vi "MAIN_CALLED_leerQR.vi"(8 "Error In":errorcluster, 11 "VISA resource name out":refnum<visa-resource-name>) -> (0 "Error Out":errorcluster)   [LabVIEW 2019]
uses:
  LVPROJ_CONFIG_ESTACION/Type_defs/Coordenadas_estacion.ctl
  LVPROJ_CREAR BANDEJAS/Type_defs/Data_Bandeja.ctl
  TYPE'S DEF/INPUT LECTURA_QR.ctl
  TYPE'S DEF/OUTPUTS_lecturaQR.ctl
  TYPE'S DEF/State_QR.ctl
  LVPROJ_MOVIMIENTO_CABEZAL/LABVIEW_MOVIMIENTO/MOVIMIENTO CABEZAL/Typedefs/Comandos.ctl
  LVPROJ_MOVIMIENTO_CABEZAL/LABVIEW_MOVIMIENTO/MOVIMIENTO CABEZAL/Typedefs/Estados_arduino.ctl
  <vilib>/Utility/error.llb/Error Cluster From Error Code.vi
  <vilib>/ErrorRing/Error Ring.xnode
  SHARED VI'S/SHARED VI'S.lvlib
panel:
  out "celda de comienzo leída":string
  out "datos leídos estacion":string
  out "trama datos enviada":string
  out "código leído?":bool
  out "read buffer 2":string
  out "caracter leido":string
  out "read buffer 3":string
  in  "Tab Control":T1(tab)
  in  "ENVIAR PARAMETROS DE LECTURA":bool
  in  "EXIT":bool
  in  "COMENZAR LECTURA":bool
  in  "LECTURA QR INPUT":T2={"COORD X"=0, "COORD  Y"=0, "NºASICS"=1, "SELECCIÓN DE BANDEJA"=enum."BANDEJA ENTRADA", "CONTEO QR"=0}
  out "INDICADORES DE TEST":T3
  out "EStado fsm":T4
  out "Configuracion Estación":T5={"Coordenadas_estacion"={"Coord.Bandeja entrada"={"Coord. X0 entrada"=0, "Coord. Y0 entrada "=0, "Altura Z entrada"=0}, "Coord.Bandeja OK"={"Coord. X0 OK"=0, "Coord. Y0 OK"=0, "Altura Z OK"=0}, "Coord.Bandeja entrada FAIL"={"Coord. X0 FAIL"=0, "Coord. Y0 FAIL"=0, "Altura Z FAIL"=0}, "Coord. Socket"={"Coord. X socket"=0, "Coord. Y socket"=0, "Altura Z socket"=0}}, "Nombre Bandeja"="", "Datos bandeja"={"Nº de columnas "=0, "Nº de filas "=0, "largo"=0, "ancho"=0, "nombre"="nombre", "Paso X (en mm)"=0.0, "Paso Y (en mm)"=0.0, "DISTANCIA SUELO A CHIP  "=0.0, "Nº de celdas totales"=0, "Distancia chips bandejas contiguas"=0.0}}
  out "FINAL QR?":bool
  out "QR pendientes":u32
  # "CELDA DE COMIENZO"
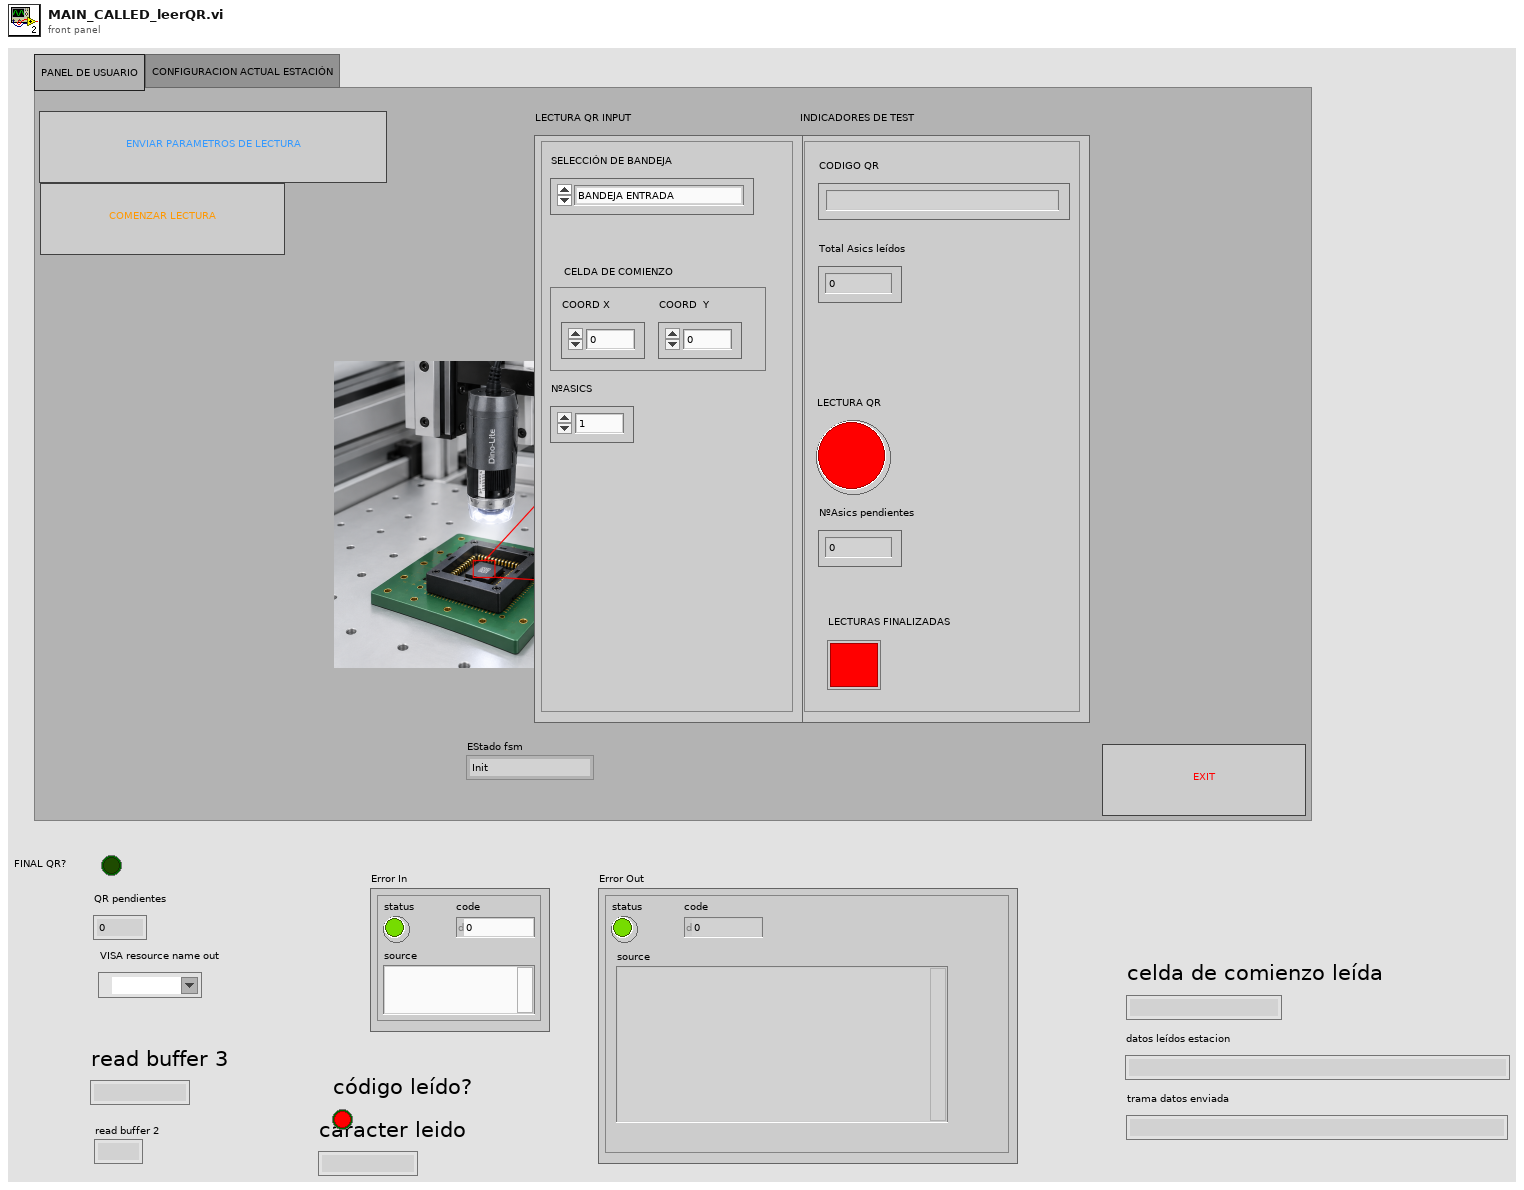
[diagram p1: front panel]
types:
  T1 = enum32{"PANEL DE USUARIO", "CONFIGURACION ACTUAL ESTACIÓN"}
  T2 = typedef "INPUT LECTURA_QR.ctl" = cluster{"COORD X":u16, "COORD  Y":u16, "NºASICS":u32, "SELECCIÓN DE BANDEJA":enum16{"BANDEJA ENTRADA", "BANDEJA OK", "BANDEJA NOK"}, "CONTEO QR":u32}
  T3 = typedef "OUTPUTS_lecturaQR.ctl" = cluster{"CODIGO QR":string, "LECTURA QR":bool, "LECTURAS FINALIZADAS":bool, "Total Asics leídos":u32, "NºAsics pendientes":u32}
  T4 = typedef "State_QR.ctl" = enum16{"Init", "Wait for Event", "Init refs", "Init com", "Config estacion", "Home", "Ping_Arduino", "Coge Asic", "Enviar_config_test", "Dejar Asic", "Leer QR", "Actualizar valores", "Enviar OK Arduino", "Final de lecturas?", "Terminar", "Exit", "Error?"}
  T5 = typedef "Configuracion_estación.ctl" = cluster{"Coordenadas_estacion":T6, "Nombre Bandeja":string, "Datos bandeja":T7}
  T6 = typedef "Coordenadas_estacion.ctl" = cluster{"Coord.Bandeja entrada":cluster{"Coord. X0 entrada":u32, "Coord. Y0 entrada ":u32, "Altura Z entrada":u32}, "Coord.Bandeja OK":cluster{"Coord. X0 OK":u32, "Coord. Y0 OK":u32, "Altura Z OK":u32}, "Coord.Bandeja entrada FAIL":cluster{"Coord. X0 FAIL":u32, "Coord. Y0 FAIL":u32, "Altura Z FAIL":u32}, "Coord. Socket":cluster{"Coord. X socket":u32, "Coord. Y socket":u32, "Altura Z socket":u32}}
  T7 = typedef "Data_Bandeja.ctl" = cluster{"Nº de columnas ":u32, "Nº de filas ":u32, "largo":u32, "ancho":u32, "nombre":string, "Paso X (en mm)":dbl, "Paso Y (en mm)":dbl, "DISTANCIA SUELO A CHIP  ":dbl, "Nº de celdas totales":u16, "Distancia chips bandejas contiguas":dbl}
  T8 = typedef "Comandos.ctl" = enum16{"H", "FH", "FM", "FI", "FX", "FY", "FZ", "I", "OK"}
  T9 = typedef "Estados_arduino.ctl" = enum16{"2", "3", "4", "5", "6", "7", "9", "8"}
  T10 = enum16{"BANDEJA ENTRADA", "BANDEJA OK", "BANDEJA NOK"}
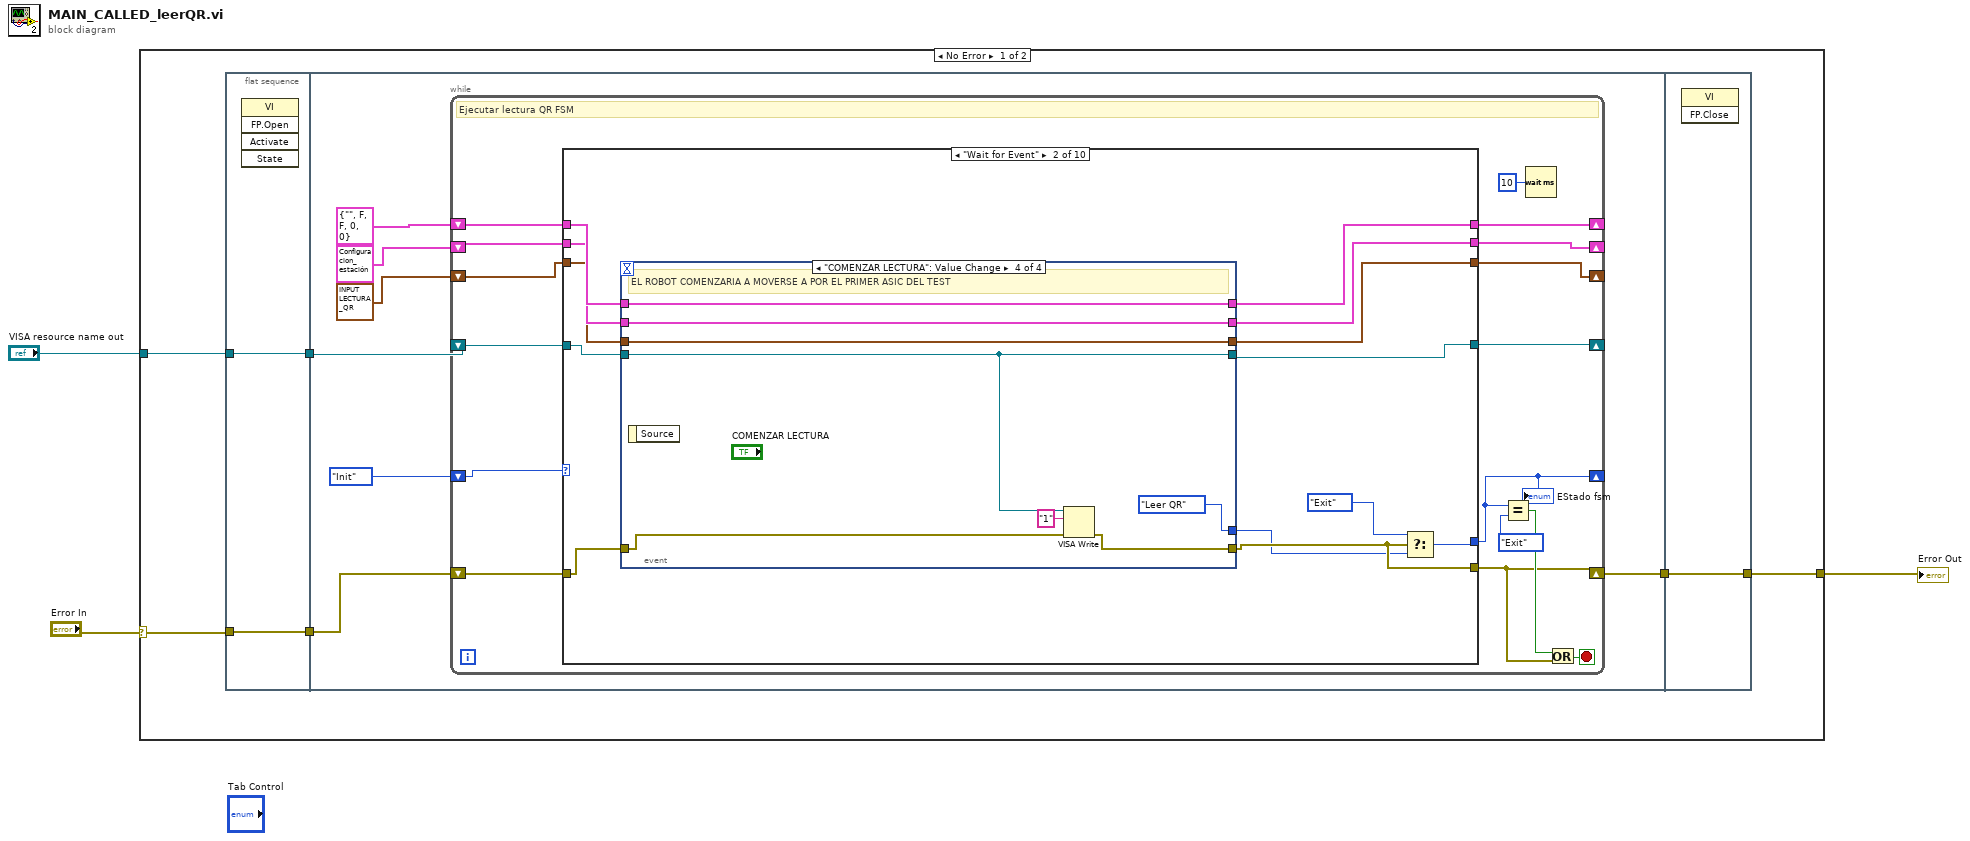
[diagram p0: block diagram]
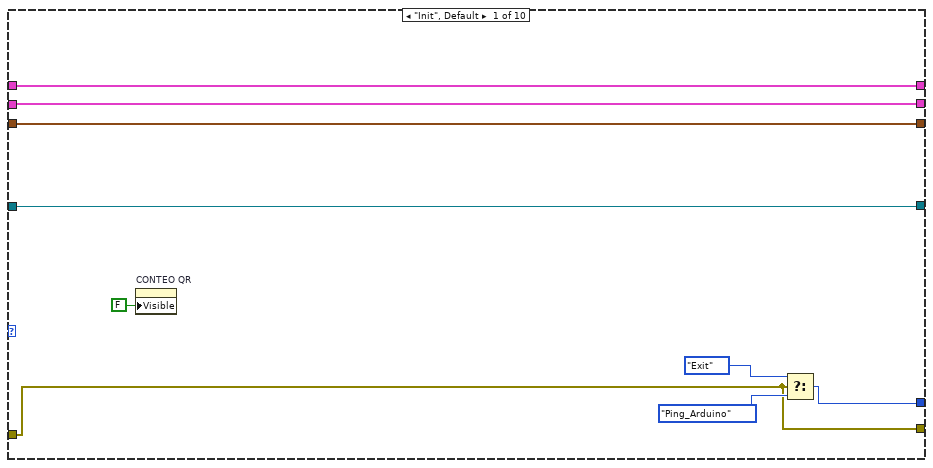
[diagram p2: hidden frame]
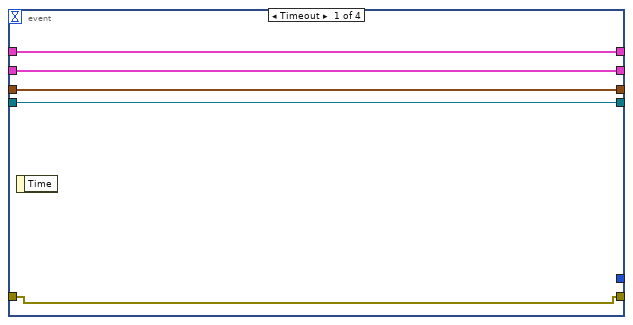
[diagram p3: hidden frame]
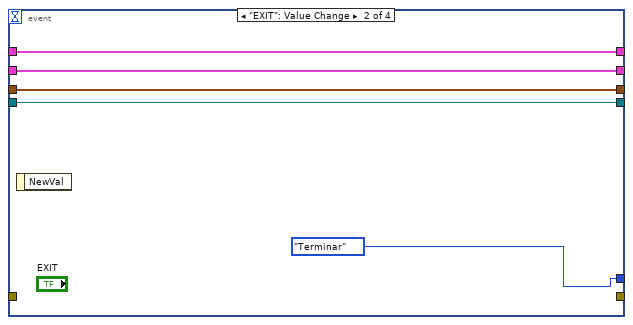
[diagram p4: hidden frame]
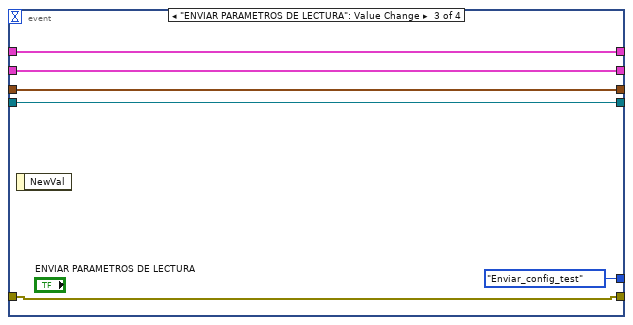
[diagram p5: hidden frame]
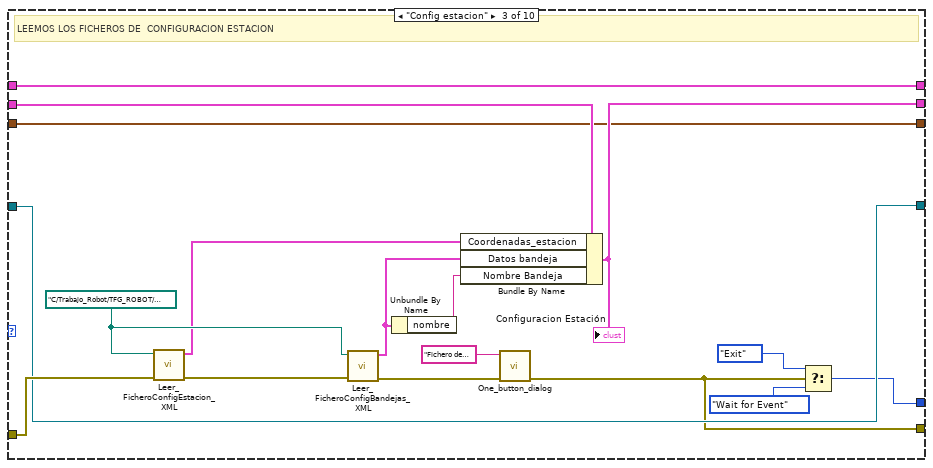
[diagram p6: hidden frame]
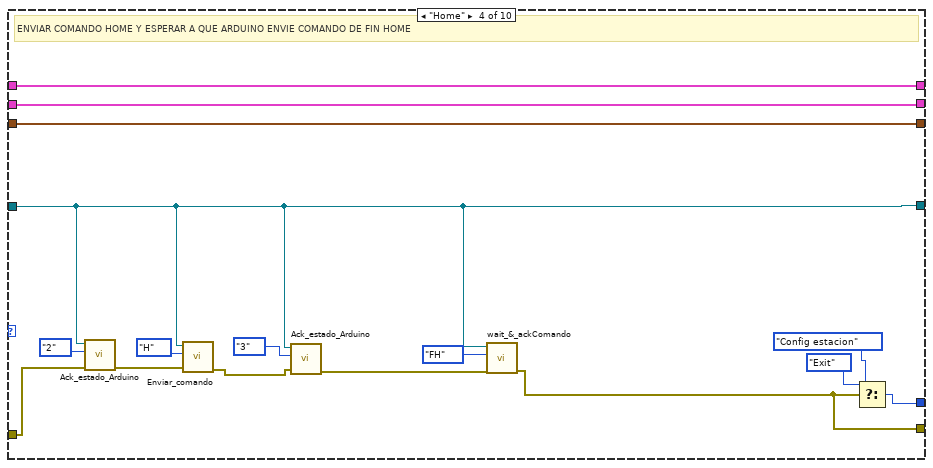
[diagram p7: hidden frame]
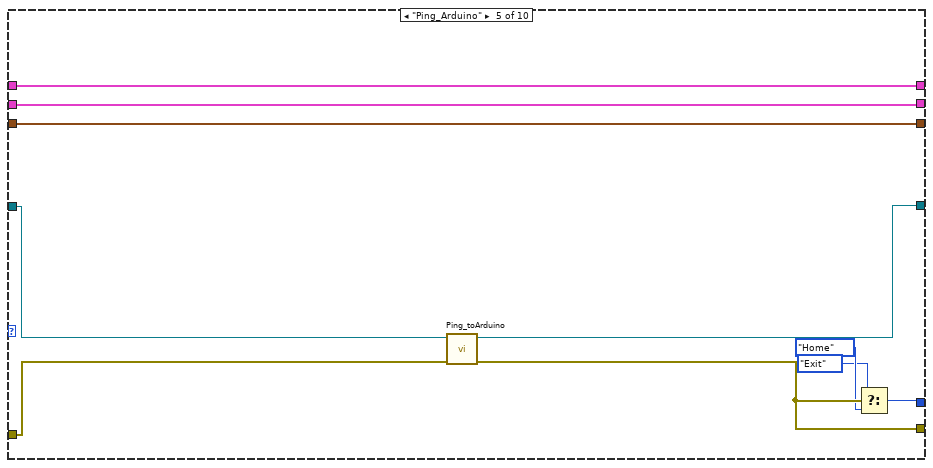
[diagram p8: hidden frame]
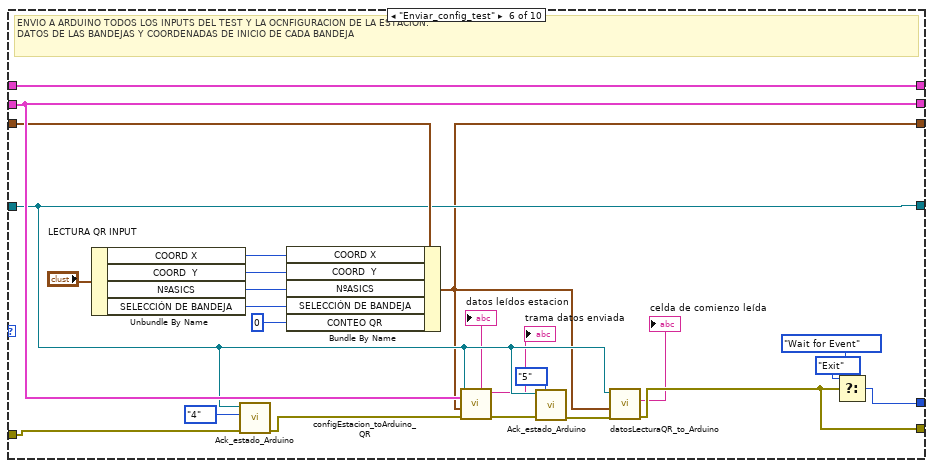
[diagram p9: hidden frame]
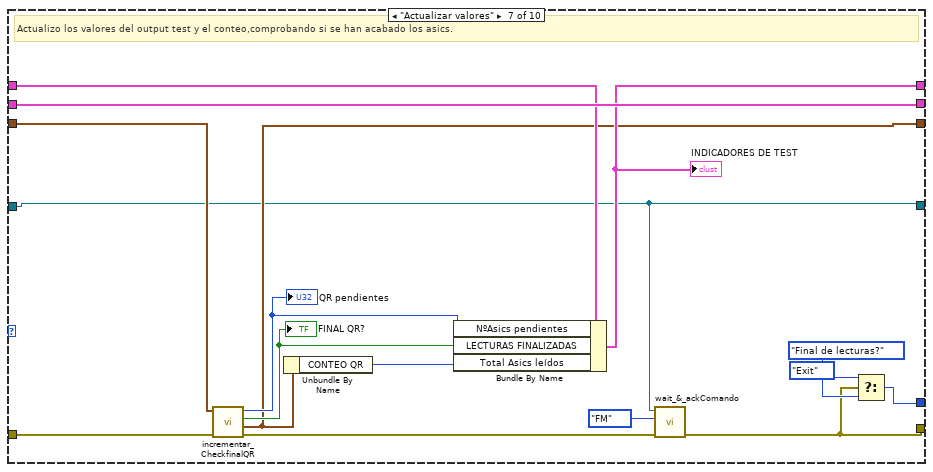
[diagram p10: hidden frame]
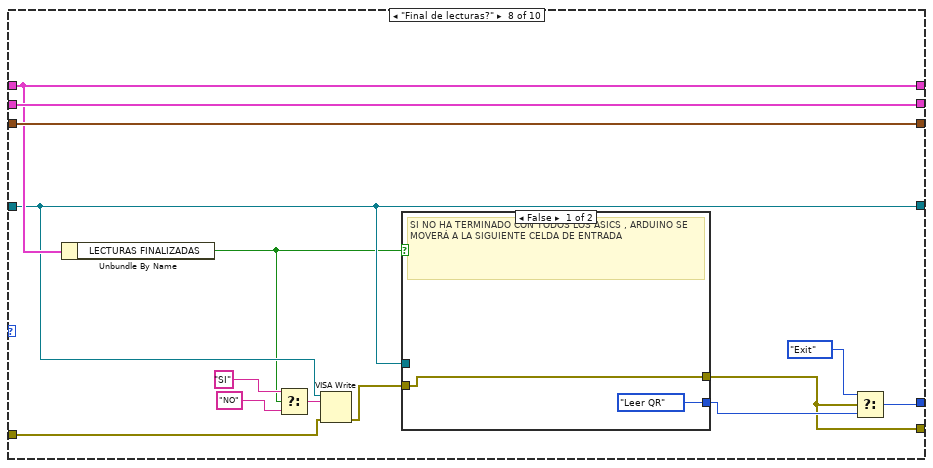
[diagram p11: hidden frame]
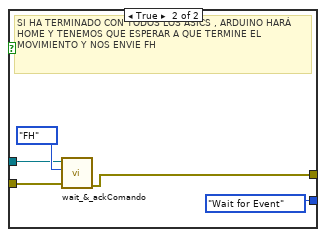
[diagram p12: hidden frame]
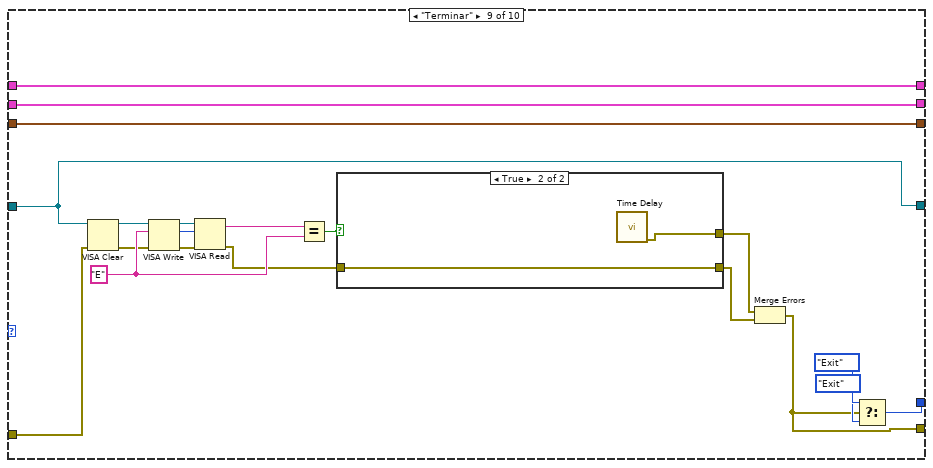
[diagram p13: hidden frame]
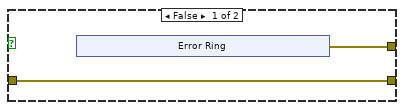
[diagram p14: hidden frame]
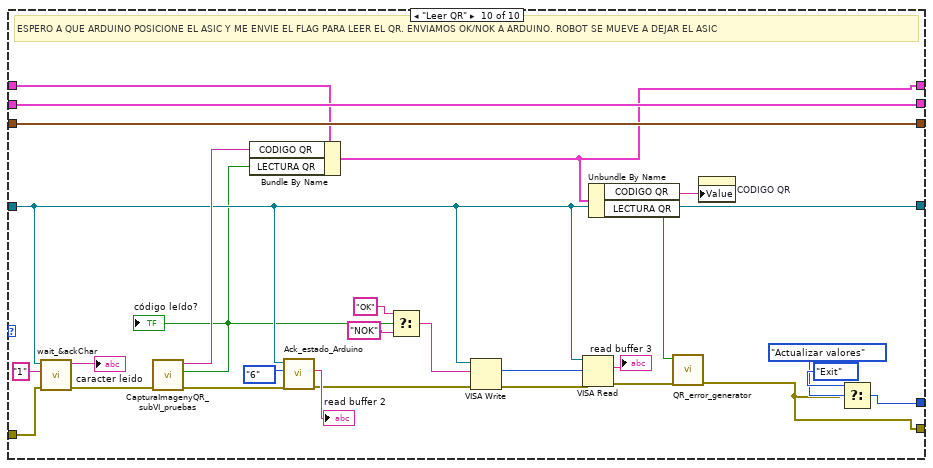
[diagram p15: hidden frame]
diagram:
  n1 = case shown="No Error" "Error In" {
    selector: "Error In" -> [w4 w243]
    tunnel: "VISA resource name out" -> [w6 _]
    tunnel: [w5 w243] -> w2
    frame No Error {
      n2 = flat-sequence {
        tunnel: w4 -> [w11]
        tunnel: [w11] -> w9
        tunnel: w6 -> [w10]
        tunnel: [w10] -> w8
        tunnel: w9 -> [w16]
        tunnel: w8 -> [w13]
        tunnel: [w12] -> w7
        tunnel: w7 -> [w242]
        tunnel: [w242] -> w5
        frame #0 {
          n3 = invoke class="VI" method="FP.Open"() -> ()  [unwired: 5 in, 5 out]
        }
        frame #1 {
          n4 = while {
            shift-right: [w29] -> w12
            shift-left: w16 -> [w33]
            shift-right: [w22] -> _
            shift-left: T2 {"COORD X"=0, "COORD  Y"=0, "NºASICS"=0, "SELECCIÓN DE BANDEJA"=enum."BANDEJA ENTRADA", "CONTEO QR"=0} ("TEST ASICS INPUT") -> [w32]
            shift-right: [w24] -> _
            shift-left: T5 {"Coordenadas_estacion"={"Coord.Bandeja entrada"={"Coord. X0 entrada"=0, "Coord. Y0 entrada "=0, "Altura Z entrada"=0}, "Coord.Bandeja OK"={"Coord. X0 OK"=0, "Coord. Y0 OK"=0, "Altura Z OK"=0}, "Coord.Bandeja entrada FAIL"={"Coord. X0 FAIL"=0, "Coord. Y0 FAIL"=0, "Altura Z FAIL"=0}, "Coord. Socket"={"Coord. X socket"=0, "Coord. Y socket"=0, "Altura Z socket"=0}}, "Nombre Bandeja"="", "Datos bandeja"={"Nº de columnas "=0, "Nº de filas "=0, "largo"=0, "ancho"=0, "nombre"="nombre", "Paso X (en mm)"=0.0, "Paso Y (en mm)"=0.0, "DISTANCIA SUELO A CHIP  "=0.0, "Nº de celdas totales"=0, "Distancia chips bandejas contiguas"=0.0}} ("Configuracion Estación") -> [w28]
            shift-right: [w26] -> _
            shift-left: w13 -> [w27]
            shift-right: [w23] -> _
            shift-left: T3 {"CODIGO QR"="", "LECTURA QR"=FALSE, "LECTURAS FINALIZADAS"=FALSE, "Total Asics leídos"=0, "NºAsics pendientes"=0} -> [w25]
            shift-right: [w20] -> _
            shift-left: State_QR."Init" ("States_main") -> [w21]
            stop <- w31 stop-if-true
            # "Ejecutar lectura QR FSM"
            n5 = case shown="\"Wait for Event\"" w21 {
              tunnel: w33 -> [w38 w50 w97 w105 w120 w135 w158 w170 w190 w241]
              tunnel: w32 -> [w36 w52 w86 w111 w121 w142 w159 w176 w202 w237]
              tunnel: [w38 w49 w82 w98 w118 w143 w150 w167 w186 w215] -> w29
              tunnel: w28 -> [w40 w54 w89 w112 w122 w144 w161 w177 w203 w238]
              tunnel: w27 -> [w39 w45 w90 w100 w119 w130 w149 w165 w189 w226]
              tunnel: [w39 w44 w90 w100 w117 w130 w149 w165 w189 w226] -> w26
              tunnel: w25 -> [w41 w56 w87 w113 w123 w145 w153 w175 w204 w233]
              tunnel: [w40 w53 w88 w112 w122 w144 w161 w177 w203 w238] -> w24
              tunnel: [w41 w55 w87 w113 w123 w145 w152 w175 w204 w232] -> w23
              tunnel: [w36 w51 w86 w111 w121 w128 w151 w176 w202 w237] -> w22
              tunnel: [w37 w46 w83 w102 w114 w136 w160 w166 w199 w236] -> w20
              frame "Init", Default {
                n6 = property on="CONTEO QR" class="DigNum (strict)"("Visible"=FALSE) -> ()  [unwired: 2 in, 2 out]
                n7 = Select(t=State_QR."Exit" ("States_main"), s=w38, f=State_QR."Ping_Arduino" ("States_main")) -> (s? t:f=w37:T4)
              }
              frame "Wait for Event" {
                n8 = event shown="[3] \"COMENZAR LECTURA\": Value Change" {
                  selector: _ -> [_ _ _ _]
                  dyn-events: _ -> [_ _ _ _]
                  timeout: _ -> [_ _ _ _]
                  tunnel: w56 -> [w61 w66 w72 w80]
                  tunnel: [w61 w66 w72 w80] -> w55
                  tunnel: w54 -> [w60 w65 w71 w79]
                  tunnel: [w60 w65 w71 w79] -> w53
                  tunnel: w52 -> [w59 w64 w70 w78]
                  tunnel: [w59 w64 w70 w78] -> w51
                  tunnel: w50 -> [w58 _ w69 w75]
                  tunnel: [w58 _ w69 w74] -> w49
                  tunnel: [_ State_QR."Terminar" ("States_main") State_QR."Enviar_config_test" ("States_main") State_QR."Leer QR" ("States_main")] -> w47
                  tunnel: w45 -> [w57 w62 w67 w76]
                  tunnel: [w57 w62 w67 w76] -> w44
                  event Timeout {
                    n9 = event-data() -> ()  [unwired: 1 in, 1 out]
                  }
                  event "EXIT": Value Change {
                    n10 = event-data() -> ()  [unwired: 1 in, 1 out]
                  }
                  event "ENVIAR PARAMETROS DE LECTURA": Value Change {
                    n11 = event-data() -> ()  [unwired: 1 in, 1 out]
                  }
                  event "COMENZAR LECTURA": Value Change {
                    # "EL ROBOT COMENZARIA A MOVERSE A POR EL PRIMER ASIC DEL TEST"
                    n12 = event-data() -> ()  [unwired: 1 in, 1 out]
                    n13 = VISA Write(VISA resource name=w76, write buffer="1", error in (no error)=w75) -> (error out=w74:errorcluster)  [unwired: 2 out]
                  }
                }
                n14 = Select(t=State_QR."Exit" ("States_main"), s=w49, f=w47) -> (s? t:f=w46:T4)
              }
              frame "Config estacion" {
                w95 = path "C:/Trabajo_Robot/TFG_ROBOT/CONTROL_ROBOT/LABVIEW_ROBOT_MASTER" ("XML File Path")
                # "LEEMOS LOS FICHEROS DE  CONFIGURACION ESTACION"
                n15 = call "Leer_FicheroConfigEstacion_XML.vi"("error in (no error)"=w97, "XML File Path"=w95) -> ("error out"=w96:errorcluster, "Coordenadas_estacion"=w94:T6)  [unwired: 8 in]
                n16 = call "Leer_FicheroConfigBandejas_XML.vi"("error in (no error)"=w96, "XML File Path"=w95) -> ("error out"=w91:errorcluster, "Datos bandeja"=w93:T7)  [unwired: 8 in]
                n17 = Unbundle By Name(w93) -> ("nombre"=w92:string)
                n18 = Bundle By Name(cluster=w89, "Coordenadas_estacion"=w94, "Datos bandeja"=w93, "Nombre Bandeja"=w92) -> (w88:T5)
                "Configuracion Estación" <- w88
                n19 = call "One_button_dialog.vi"("error in (no error)"=w91, "message"="Fichero de configuración cargado correctamente.") -> ("error out"=w82:errorcluster)  [unwired: 9 in]
                n20 = Select(t=State_QR."Exit" ("States_main"), s=w82, f=State_QR."Wait for Event" ("States_main")) -> (s? t:f=w83:T4)
              }
              frame "Home" {
                # "ENVIAR COMANDO HOME Y ESPERAR A QUE ARDUINO ENVIE COMANDO DE FIN HOME"
                n21 = call "Ack_estado_Arduino.vi"("error in (no error)"=w105, "Enum"=Estados_arduino."2", "VISA resource name"=w100) -> ("error out"=w110:errorcluster)  [unwired: 6 in, 2 out]
                n22 = call "Enviar_comando.vi"("error in (no error)"=w110, "Enum"=Comandos."H", "VISA resource name"=w100) -> ("error out"=w106:errorcluster)  [unwired: 6 in, 2 out]
                n23 = call "Ack_estado_Arduino.vi"("error in (no error)"=w106, "Enum"=Estados_arduino."3", "VISA resource name"=w100) -> ("error out"=w101:errorcluster)  [unwired: 6 in, 2 out]
                n24 = call "wait_&_ackComando.vi"("error in (no error)"=w101, 10:Comandos."FH", "VISA Refnum in"=w100) -> ("error out"=w98:errorcluster)  [unwired: 7 in, 1 out]
                n25 = Select(t=State_QR."Exit" ("States_main"), s=w98, f=State_QR."Config estacion" ("States_main")) -> (s? t:f=w102:T4)
              }
              frame "Ping_Arduino" {
                n26 = call "Ping_toArduino.vi"("error in (no error)"=w120, "VISA Refnum in"=w119) -> ("error out"=w118:errorcluster, "VISA Refnum out"=w117:refnum<visa-resource-name>)  [unwired: 7 in, 1 out]
                n27 = Select(t=State_QR."Exit" ("States_main"), s=w118, f=State_QR."Home" ("States_main")) -> (s? t:f=w114:T4)
              }
              frame "Enviar_config_test" {
                # "ENVIO A ARDUINO TODOS LOS INPUTS DEL TEST Y LA OCNFIGURACION DE LA ESTACIÓN:\nDATOS DE LAS BANDEJAS Y COORDENADAS DE INICIO DE CADA BANDEJA"
                n28 = Unbundle By Name("LECTURA QR INPUT") -> ("COORD X"=w141:u16, "COORD  Y"=w140:u16, "NºASICS"=w139:u32, "SELECCIÓN DE BANDEJA"=w138:T10)
                n29 = call "Ack_estado_Arduino.vi"("error in (no error)"=w135, "Enum"=Estados_arduino."4", "VISA resource name"=w130) -> ("error out"=w133:errorcluster)  [unwired: 6 in, 2 out]
                n30 = Bundle By Name(cluster=w142, "COORD X"=w141, "COORD  Y"=w140, "NºASICS"=w139, "SELECCIÓN DE BANDEJA"=w138, "CONTEO QR"=u32 0) -> (w128:T2)
                n31 = call "configEstacion_toArduino_QR.vi"("error in (no error)"=w133, "LECTURA QR INPUT"=w128, "Configuracion Estación"=w144, "VISA resource name"=w130) -> ("error IO"=w132:errorcluster, "datos leídos"=→"datos leídos estacion":string, "trama datos enviada"=→"trama datos enviada":string)  [unwired: 5 in]
                n32 = call "Ack_estado_Arduino.vi"("error in (no error)"=w132, "Enum"=Estados_arduino."5", "VISA resource name"=w130) -> ("error out"=w131:errorcluster)  [unwired: 6 in, 2 out]
                n33 = call "datosLecturaQR_to_Arduino.vi"("error in (no error)"=w131, "LECTURA QR INPUT"=w128, "VISA resource name"=w130) -> ("error IO"=w143:errorcluster, "celda de comienzo leída"=→"celda de comienzo leída":string)  [unwired: 7 in]
                n34 = Select(t=State_QR."Exit" ("States_main"), s=w143, f=State_QR."Wait for Event" ("States_main")) -> (s? t:f=w136:T4)
              }
              frame "Actualizar valores" {
                # "Actualizo los valores del output test y el conteo,comprobando si se han acabado los asics."
                n35 = call "incrementar_CheckfinalQR.vi"("error in (no error)"=w158, "TEST ASICS INPUT"=w159) -> ("error out"=w157:errorcluster, "output cluster"=w151:T2, "FINAL ASICS??"=w155:bool, "Asics pendientes"=w156:u32)  [unwired: 6 in]
                "FINAL QR?" <- w155
                "QR pendientes" <- w156
                n36 = Unbundle By Name(w151) -> ("CONTEO QR"=w154:u32)
                n37 = Bundle By Name(cluster=w153, "NºAsics pendientes"=w156, "LECTURAS FINALIZADAS"=w155, "Total Asics leídos"=w154) -> (w152:T3)
                "INDICADORES DE TEST" <- w152
                n38 = call "wait_&_ackComando.vi"("error in (no error)"=w157, 10:Comandos."FM", "VISA Refnum in"=w149) -> ("error out"=w150:errorcluster)  [unwired: 7 in, 1 out]
                n39 = Select(t=State_QR."Exit" ("States_main"), s=w150, f=State_QR."Final de lecturas?" ("States_main")) -> (s? t:f=w160:T4)
              }
              frame "Final de lecturas?" {
                n40 = Unbundle By Name(w175) -> ("LECTURAS FINALIZADAS"=w164:bool)
                n41 = Select(t="SI", s=w164, f="NO") -> (s? t:f=w172:string)
                n42 = VISA Write(VISA resource name=w165, write buffer=w172, error in (no error)=w170) -> (error out=w171:errorcluster)  [unwired: 2 out]
                n43 = case shown="False" w164 {
                  tunnel: w171 -> [w179 w184]
                  tunnel: [w179 w182] -> w167
                  tunnel: [State_QR."Leer QR" ("States_main") State_QR."Wait for Event" ("States_main")] -> w169
                  tunnel: w165 -> [_ w180]
                  frame False {
                    # "SI NO HA TERMINADO CON TODOS LOS ASICS , ARDUINO SE MOVERÁ A LA SIGUIENTE CELDA DE ENTRADA"
                  }
                  frame True {
                    # "SI HA TERMINADO CON TODOS LOS ASICS , ARDUINO HARÁ HOME Y TENEMOS QUE ESPERAR A QUE TERMINE EL MOVIMIENTO Y NOS ENVIE FH"
                    n44 = call "wait_&_ackComando.vi"("error in (no error)"=w184, 10:Comandos."FH", "VISA Refnum in"=w180) -> ("error out"=w182:errorcluster)  [unwired: 7 in, 1 out]
                  }
                }
                n45 = Select(t=State_QR."Exit", s=w167, f=w169) -> (s? t:f=w166:T4)
              }
              frame "Terminar" {
                w195 = "E" ("write buffer")
                n46 = VISA Clear(VISA resource name=w189, error in (no error)=w190) -> (VISA resource name out=w185:refnum<visa-resource-name>, error out=w191:errorcluster)
                n47 = VISA Write(VISA resource name=w185, write buffer=w195, error in (no error)=w191) -> (VISA resource name out=w198:refnum<visa-resource-name>, return count=w197:u32, error out=w192:errorcluster)
                n48 = VISA Read(VISA resource name=w198, byte count=w197, error in (no error)=w192) -> (read buffer=w196:string, error out=w188:errorcluster)  [unwired: 2 out]
                n49 = Equal?(x=w196, y=w195) -> (x = y?=w194:bool)
                n50 = case shown="True" w194 {
                  tunnel: [w206 w213] -> w193
                  tunnel: w188 -> [w205 w212]
                  tunnel: [w205 w212] -> w187
                  frame False {
                    n51 = xnode "Error Ring"() -> ("error out"=w206:errorcluster)
                  }
                  frame True {
                    n52 = call "Time Delay"() -> ("error out"=w213:errorcluster)  [unwired: 11 in]
                  }
                }
                n53 = Merge Errors(w193, w187) -> (w186:errorcluster)
                n54 = Select(t=State_QR."Exit" ("y"), s=w186, f=State_QR."Exit" ("y")) -> (s? t:f=w199:T4)
              }
              frame "Leer QR" {
                # "ESPERO A QUE ARDUINO POSICIONE EL ASIC Y ME ENVIE EL FLAG PARA LEER EL QR. ENVIAMOS OK/NOK A ARDUINO. ROBOT SE MUEVE A DEJAR EL ASIC"
                n55 = call "wait_&ackChar.vi"("error in (no error)"=w241, "caracter"="1", "VISA Refnum in"=w226) -> ("error out"=w230:errorcluster, "caracter leido"=→"caracter leido":string)  [unwired: 7 in]
                n56 = call "CapturaImagenyQR_subVI_pruebas.vi"("error in (no error)"=w230) -> ("error out"=w222:errorcluster, "código leído?"=w221:bool, "Datos_QR"=w234:string)  [unwired: 8 in]
                "código leído?" <- w221
                n57 = Bundle By Name(cluster=w233, "CODIGO QR"=w234, "LECTURA QR"=w221) -> (w232:T3)
                n58 = call "Ack_estado_Arduino.vi"("error in (no error)"=w222, "Enum"=Estados_arduino."6", "VISA resource name"=w226) -> ("error out"=w214:errorcluster, "read buffer"=→"read buffer 2":string)  [unwired: 6 in, 1 out]
                n59 = Select(t="OK" ("write buffer"), s=w221, f="NOK") -> (s? t:f=w218:string)
                n60 = VISA Write(VISA resource name=w226, write buffer=w218, error in (no error)=w214) -> (return count=w227:u32, error out=w225:errorcluster)  [unwired: 1 out]
                n61 = VISA Read(VISA resource name=w226, byte count=w227, error in (no error)=w225) -> (read buffer=→"read buffer 3":string, error out=w216:errorcluster)  [unwired: 2 out]
                n62 = Unbundle By Name(w232) -> ("CODIGO QR"=w231:string, "LECTURA QR"=w217:bool)
                n63 = call "QR_error_generator.vi"("Error In"=w216, "CODIGO QR LEÍDO?"=w217) -> ("Error Out"=w215:errorcluster)  [unwired: 9 in]
                n64 = property on="CODIGO QR" class="Str"("Value"=w231) -> ()  [unwired: 2 in, 2 out]
                n65 = Select(t=State_QR."Exit" ("States_main"), s=w215, f=State_QR."Actualizar valores" ("States_main")) -> (s? t:f=w236:T4)
              }
            }
            "EStado fsm" <- w20
            n66 = Equal?(x=w20, y=State_QR."Exit") -> (x = y?=w34:bool)
            n67 = Wait (ms)(milliseconds to wait=u32 10) -> ()  [unwired: 1 out]
            n68 = Or(x=w34, y=w29) -> (x .or. y?=w31:bool)
          }
        }
        frame #2 {
          n69 = invoke class="VI" method="FP.Close"() -> ()  [unwired: 3 in, 3 out]
        }
      }
    }
    frame Error {
    }
  }
  "Error Out" <- w2
